vi "lab_2_thermistor_sensor.vi"(1 "voltage":dbl) -> (0 "temp_celsius":dbl)   [LabVIEW 2020]
uses:
  <vilib>/imath/engines/lvmath2/RunTimeEngine/Managers/WorkSpace/UID Generator.vi
  <vilib>/imath/engines/lvmath2/RunTimeEngine/RunTimeType/NIMS_RunTimeType_From StrictType (excl LVString).vi
  <instcachedir>/0/NIMS_RunTimeType_From StrictType (excl LVString)_283B1B2000484AAA8744D21CE97EA49F.lvgen/NIMS_RunTimeType_From StrictType (excl LVString)_283B1B2000484AAA8744D21CE97EA49F_000.vi
  <vilib>/imath/engines/lvmath2/RunTimeEngine/LocalVariableDefStatement/MC_LocalVariableDefStatement_Display.vi
  <vilib>/imath/engines/lvmath2/RunTimeEngine/BuiltInFunctions/power/NIMS_power.vi
  <instcachedir>/0/NIMS_power_74787A1A750E429FBFF382073624D570.lvgen/NIMS_power_74787A1A750E429FBFF382073624D570_011.vi
  <vilib>/imath/engines/lvmath2/RunTimeEngine/Managers/SymbolTable/Clear UID.vi
  <vilib>/imath/engines/lvmath2/RunTimeEngine/NodeEndStatement/NIMS_NodeEndStatement_Output.vi
  <instcachedir>/0/NIMS_NodeEndStatement_Output_53EC0D466D134D7ABD903AC30B43404B.lvgen/NIMS_NodeEndStatement_Output_53EC0D466D134D7ABD903AC30B43404B_009.vi
  <vilib>/imath/engines/lvmath2/RunTimeEngine/ErrorHandling/NIMS_Finalize Error.vi
  <vilib>/imath/engines/lvmath2/RunTimeEngine/Managers/SymbolTable/NIMS_WorkSpace.lvlib
panel:
  out "temp_kelvin":dbl
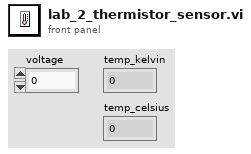
[diagram p1: front panel]
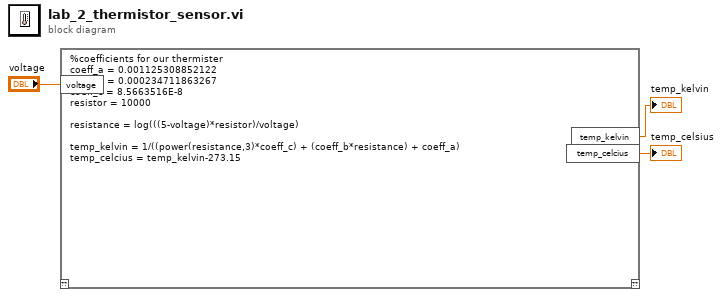
[diagram p0: block diagram]
diagram:
  n1 = mathscript code="%coefficients for our thermister\ncoeff_a = 0.001125308852122\ncoeff_b = 0.000234711863267\ncoeff_c = 8.5663516E-8\nresistor = 10000\n\nresistance = log(((5-voltage)*resistor)/voltage)\n\ntemp_kelvin = 1/((power(resistance,3)*coeff_c) + (coeff_b*resistance) + coeff_a)\ntemp_celcius = temp_kelvin-273.15"("voltage"="voltage") -> ("temp_kelvin"=→"temp_kelvin":cdb, "temp_celcius"=→"temp_celsius":cdb)  [unwired: 1 in, 1 out]
